vi "User Events + DVRs.vi"() -> ()   [LabVIEW 2017]
doc: "Template for creation user event and DVRs for SW"
uses:
  Error Handler/Controls/Error Type.ctl
  Error Handler/Controls/Error Message.ctl
  Configuration/Controls/Config DB Command.ctl
  Configuration/Controls/Config DB Message.ctl
  Configuration/Controls/Config DB Record1.ctl
  Configuration/Controls/Config DB Overhead.ctl
  Views/Vehicle Position Simulation View/Controls/Vehicle - Position.ctl
  Controller/Controls/Controller Overhead.ctl
  Controller/Controls/Controller Wash Step.ctl
  Model/Controls/Views Action.ctl
  Controller/Controls/Controller State.ctl
panel:
  in  "Views Command":refnum<user-event>
  in  "Out Of Position":refnum<user-event>
  in  "Wash Step Start":refnum<user-event>
  in  "Views Action":refnum<user-event>
  in  "Start Wash":refnum<user-event>
  in  "Overhead DVR":refnum<data-value>
  in  "Position Change":refnum<user-event>
  in  "Config DVR":refnum<data-value>
  in  "Config":refnum<user-event>
  in  "Error":refnum<user-event>
  in  "Stop DVR":refnum<data-value>
  in  "Stop":refnum<user-event>
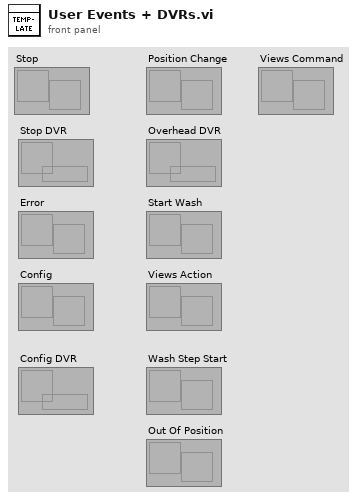
[diagram p1: front panel]
types:
  T1 = typedef "Controller State.ctl" = enum16{"Initial", "Wait for Start", "Wash Cycle Start", "Wash Cycle Complete", "Wash Step Start", "Wash Step Execute", "Wash Step Complete", "Wait for Vehicle Position", "Wash Exit", "Wash Abort/Terminate"}
  T2 = typedef "Controller Wash Step.ctl" = enum16{"None", "Under Body Wash", "Bug Remover", "Pre-Soak", "High Pressure Wash", "Low Pressure Wax", "Spot Free Rinse", "Tire Shine Foam", "Air Dry"}
  T3 = typedef "Views Action.ctl" = enum16{"Initial", "Wash Cycle Start", "Wash Cycle Complete", "Wash Exit", "Wash Abort/Terminate", "Wash Step Start", "Wash Step Execute", "Wash Step Complete"}
  T4 = typedef "Controller Overhead.ctl" = cluster{"Current Position":T5, "Wash Enclosure":T2[], "Current State":T1, "Next State":T1}
  T5 = typedef "Vehicle - Position.ctl" = enum16{"Entry", "Station 1", "Station 2", "Station 3", "Exit"}
  T6 = typedef "Config DB Overhead.ctl" = cluster{"Locked DB?":bool, "DB Records Array":T7[], "Queried Step Duration":u32}
  T7 = typedef "Config DB Record1.ctl" = cluster{"Wash Step":string, "Station":string, "Step Duration":u32}
  T8 = typedef "Config DB Message.ctl" = cluster{"DB Command":T9, "DB Data":variant}
  T9 = typedef "Config DB Command.ctl" = enum16{"Read records", "Query timing", "Insert new data", "Update data", "Lock DB", "Unlock DB"}
  T10 = typedef "Error Message.ctl" = cluster{"Error Type":T11, "Error Data":variant}
  T11 = typedef "Error Type.ctl" = enum16{"Minor Error", "Wash Cycle Error", "System Error", "Unknown"}
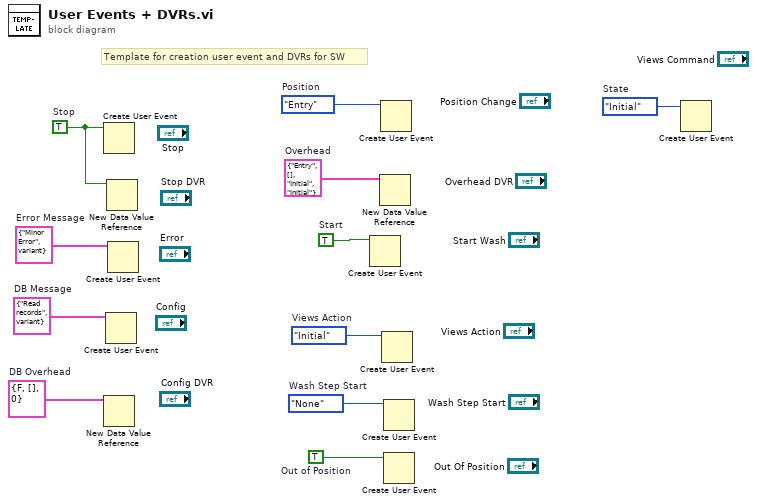
[diagram p0: block diagram]
diagram:
  w1 = Controller_State."Initial"  # State
  w2 = TRUE  # Out of Position
  w3 = Controller_Wash_Step."None"  # Wash Step Start
  w4 = Views_Action."Initial"  # Views Action
  w5 = TRUE  # Start
  w6 = T4 {"Current Position"=enum."Entry", "Wash Enclosure"=[], "Current State"=enum."Initial", "Next State"=enum."Initial"}  # Overhead
  w7 = Vehicle_-_Position."Entry"  # Position
  w8 = T6 {"Locked DB?"=FALSE, "DB Records Array"=[], "Queried Step Duration"=0}  # DB Overhead
  w9 = T8 {"DB Command"=enum."Read records", "DB Data"=variant}  # DB Message
  w10 = T10 {"Error Type"=enum."Minor Error", "Error Data"=variant}  # Error Message
  w11 = TRUE  # Stop
  # "Template for creation user event and DVRs for SW"
  n1 = Create User Event(user event datatype=w11) -> ()  [unwired: 1 in, 2 out]
  n2 = New Data Value Reference(data value=w8) -> ()  [unwired: 1 in, 2 out]
  n3 = Create User Event(user event datatype=w9) -> ()  [unwired: 1 in, 2 out]
  n4 = New Data Value Reference(data value=w11) -> ()  [unwired: 1 in, 2 out]
  n5 = Create User Event(user event datatype=w10) -> ()  [unwired: 1 in, 2 out]
  n6 = Create User Event(user event datatype=w5) -> ()  [unwired: 1 in, 2 out]
  n7 = New Data Value Reference(data value=w6) -> ()  [unwired: 1 in, 2 out]
  n8 = Create User Event(user event datatype=w7) -> ()  [unwired: 1 in, 2 out]
  n9 = Create User Event(user event datatype=w4) -> ()  [unwired: 1 in, 2 out]
  n10 = Create User Event(user event datatype=w3) -> ()  [unwired: 1 in, 2 out]
  n11 = Create User Event(user event datatype=w2) -> ()  [unwired: 1 in, 2 out]
  n12 = Create User Event(user event datatype=w1) -> ()  [unwired: 1 in, 2 out]
